vi "Log_Everything_To_Buffer.vi"(8 "error in":errorcluster, 9 "array of string values":string[](array[string]), 10 "array of doubles":dbl[](array[numeric]), 11 "Iteration/Line Number":dbl format="%#_13g") -> (0 "error out":errorcluster)   [LabVIEW 2017]
uses:
  frc-software-2018/SwerveLibrary/Huskie Swerve.lvlib
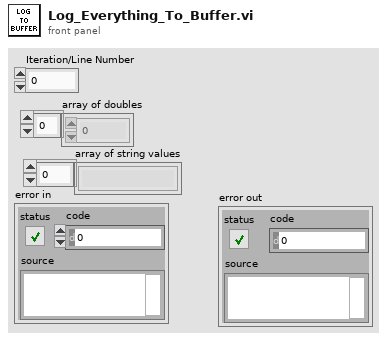
[diagram p1: front panel]
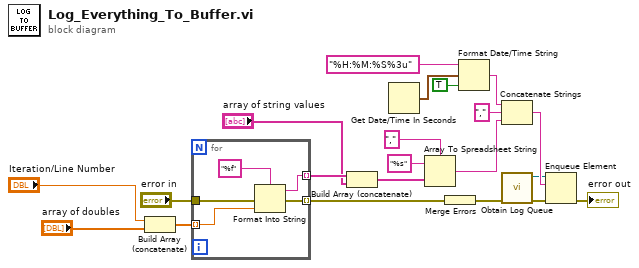
[diagram p0: block diagram]
diagram:
  n1 = Build Array (concatenate)("Iteration/Line Number", "array of doubles") -> (w19:dbl[])
  n2 = for {
    tunnel: w19 -> [w26] mode=indexing
    tunnel: [w24] -> w17 mode=indexing
    tunnel: "error in" -> [w23]
    tunnel: [w22] -> w4 mode=indexing
    n3 = Format Into String(format string="%f", error in=w23, w26) -> (resulting string=w24:string, error out=w22:errorcluster)  [unwired: 1 in]
  }
  n4 = Build Array (concatenate)(w17, "array of string values") -> (w13:string[])
  n5 = Get Date/Time In Seconds() -> (seconds since 1Jan1904=w11:timestamp)
  n6 = Array To Spreadsheet String(delimiter (Tab)=",", array=w13, 3:"%s" ("format string")) -> (spreadsheet string=w12:string)
  n7 = Merge Errors(w4) -> (w3:errorcluster)
  n8 = Format Date/Time String(time format string (%c)="%H:%M:%S%3u", seconds (now)=w11, UTC format=TRUE) -> (date/time string=w8:string)
  n9 = Concatenate Strings(w8, "," ("string"), w12) -> (w6:string)
  n10 = call "Obtain Log Queue.vi"("error in"=w3) -> ("error out"=w2:errorcluster, "queue out"=w5:refnum<queue>)  [unwired: 9 in]
  n11 = Enqueue Element(queue=w5, element=w6, error in (no error)=w2) -> (error out=→"error out":errorcluster)  [unwired: 1 in, 2 out]
